vi "Get Data.vi"(8 "error in":errorcluster, 11 "Cfg Dev in":refnum<class "Vaisala.lvclass">) -> (0 "error out":errorcluster, 2 "Data":refnum<class "Data.lvclass">, 3 "Cfg Dev out":refnum<class "Vaisala.lvclass">)   [LabVIEW 2015, in "Vaisala Library.lvlib" / "Vaisala.lvclass"]
uses:
  Vaisala.lvclass
  <vilib>/MSR Consulting, LLC/General Reuse/Session APIs/Serial/Serial Session.lvclass
  Data/Vaisala Data.lvclass
  <vilib>/MSR Consulting, LLC/General Reuse/Data/Data.lvclass
  <vilib>/MSR Consulting, LLC/General Reuse/Session APIs/Session Log/System Log.lvclass
  <vilib>/MSR Consulting, LLC/General Reuse/Session APIs/Serial/Public/Get Data/Get String.vi
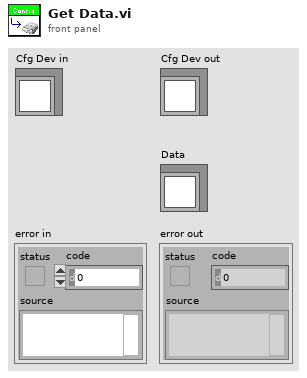
[diagram p1: front panel]
types:
  T1 = typedef "Session - Root.lvclass/Session Handle.ctl" = refnum<data-value>
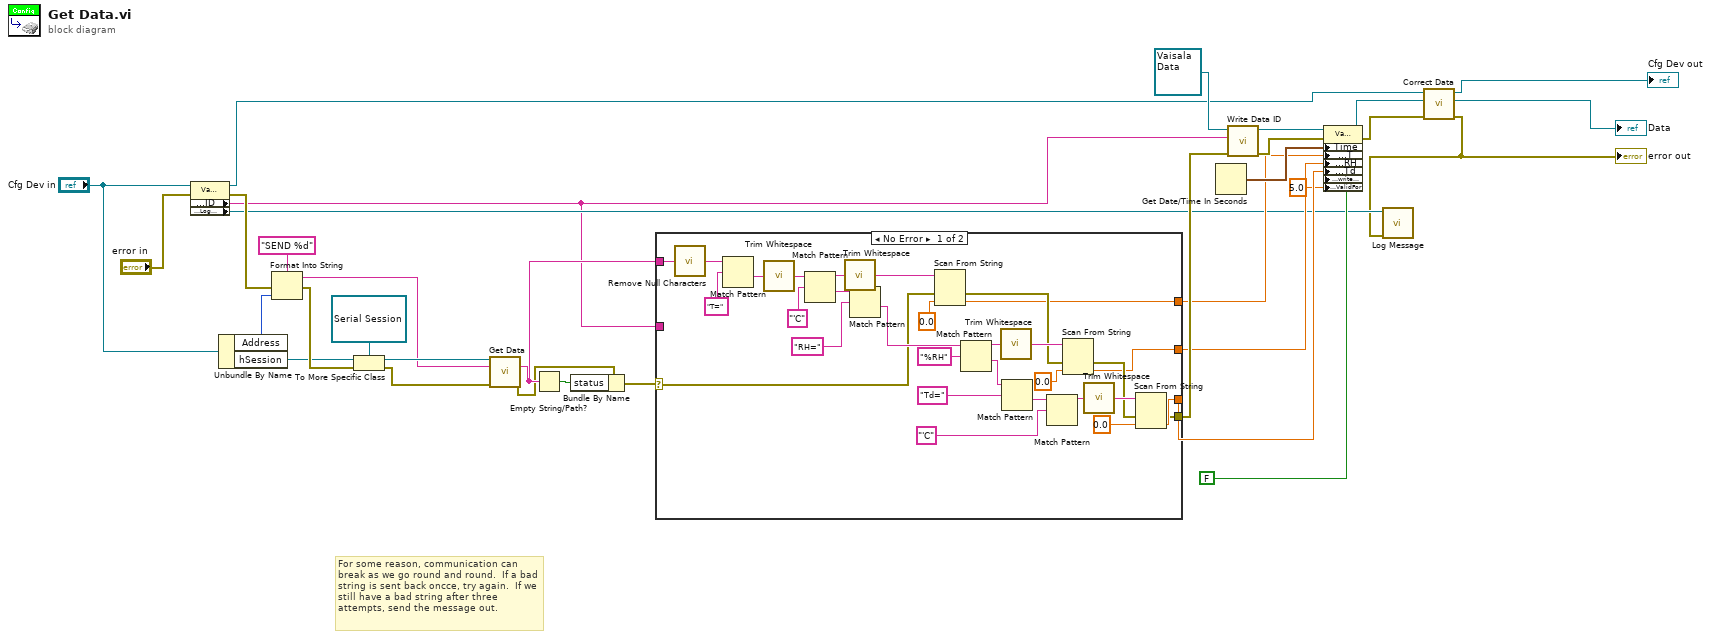
[diagram p0: block diagram]
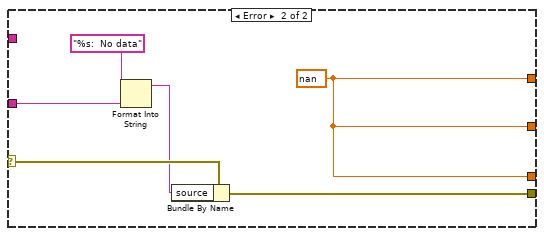
[diagram p2: hidden frame]
diagram:
  # "For some reason, communication can break as we go round and round.  If a bad string is sent back oncce, try again.  If we still have a bad string after three attempts, send the message out."
  n1 = property class="Vaisala.lvclass"(reference="Cfg Dev in", error in="error in") -> (reference out=w10:refnum<class "Vaisala.lvclass">, error out=w19:errorcluster, "Accessors:ID"=w2:string, "Accessors:Log Session"=w12:T1)
  n2 = Unbundle By Name("Cfg Dev in") -> ("Address"=w33:u8, "hSession"=w28:T1)
  n3 = Format Into String(format string="SEND %d", error in=w19, w33) -> (resulting string=w14:string, error out=w29:errorcluster)  [unwired: 1 in]
  n4 = To More Specific Class(target class=refnum<data-value> refnum ("hSession"), reference=w28, error in=w29) -> (specific class reference=w27:refnum<data-value>, error out=w26:errorcluster)
  n5 = call-poly <vilib>:"Get Data.vi"("Session Handle in"=w27, "CMD"=w14, "error in"=w26) -> ("DataOut"=w13:string, "error out"=w5:errorcluster)  [unwired: 10 in, 1 out]
  n6 = Empty String/Path?(string/path=w13) -> (empty?=w4:bool)
  n7 = Bundle By Name(cluster=w5, "status"=w4) -> (w3:errorcluster)
  n8 = case shown="No Error" w3 {
    selector: w3 -> [w34 w66]
    tunnel: [w40 w69] -> w15
    tunnel: [w39 w69] -> w16
    tunnel: [w38 w69] -> w17
    tunnel: [w37 w65] -> w18
    tunnel: w13 -> [w35 _]
    tunnel: w2 -> [_ w67]
    frame No Error {
      n9 = call <vilib>:"Remove Null Characters.vi"("String"=w35) -> ("string"=w36:string)  [unwired: 4 in]
      n10 = Match Pattern(string=w36, regular expression="T=") -> (after substring=w62:string)  [unwired: 1 in, 3 out]
      n11 = call <vilib>:"Trim Whitespace.vi"("string"=w62) -> ("trimmed string"=w61:string)  [unwired: 1 in]
      n12 = Match Pattern(string=w61, regular expression="'C") -> (before substring=w59:string, after substring=w56:string)  [unwired: 1 in, 2 out]
      n13 = call <vilib>:"Trim Whitespace.vi"("string"=w59) -> ("trimmed string"=w58:string)  [unwired: 1 in]
      n14 = Match Pattern(string=w56, regular expression="RH=") -> (after substring=w53:string)  [unwired: 1 in, 3 out]
      n15 = Scan From String(input string=w58, error in=w34, default 1=sgl 0.0 ("output 1")) -> (error out=w42:errorcluster, output 1=w38:sgl)  [unwired: 2 in, 2 out]
      n16 = Match Pattern(string=w53, regular expression="%RH") -> (before substring=w50:string, after substring=w48:string)  [unwired: 1 in, 2 out]
      n17 = call <vilib>:"Trim Whitespace.vi"("string"=w50) -> ("trimmed string"=w51:string)  [unwired: 1 in]
      n18 = Match Pattern(string=w48, regular expression="Td=") -> (after substring=w46:string)  [unwired: 1 in, 3 out]
      n19 = Match Pattern(string=w46, regular expression="'C") -> (before substring=w43:string)  [unwired: 1 in, 3 out]
      n20 = Scan From String(input string=w51, error in=w42, default 1=sgl 0.0 ("output 1")) -> (error out=w41:errorcluster, output 1=w39:sgl)  [unwired: 2 in, 2 out]
      n21 = call <vilib>:"Trim Whitespace.vi"("string"=w43) -> ("trimmed string"=w44:string)  [unwired: 1 in]
      n22 = Scan From String(input string=w44, error in=w41, default 1=sgl 0.0 ("output 1")) -> (error out=w37:errorcluster, output 1=w40:sgl)  [unwired: 2 in, 2 out]
    }
    frame Error {
      w69 = sgl nan ("output 1")
      n23 = Format Into String(format string="%s:  No data", w67) -> (resulting string=w64:string)  [unwired: 2 in, 1 out]
      n24 = Bundle By Name(cluster=w66, "source"=w64) -> (w65:errorcluster)
    }
  }
  n25 = Get Date/Time In Seconds() -> (seconds since 1Jan1904=w31:timestamp)
  n26 = call <vilib>:"Write Data ID.vi"("error in"=w18, "Data ID"=w2, "Data in"=refnum<class "Vaisala Data.lvclass"> refnum ("Vaisala Library.lvlib:Vaisala Data.lvclass")) -> ("error out"=w23:errorcluster, "Data out"=w24:refnum<class "Vaisala Data.lvclass">)  [unwired: 7 in]
  n27 = property class="Vaisala Data"(reference=w24, error in=w23, "Time"=w31, "Accessors:T"=w17, "Accessors:RH"=w16, "Accessors:Td"=w15, "Accessors:write time"=FALSE ("write time"), "Accessors:ValidFor"=5.0 ("ValidFor")) -> (reference out=w9:refnum<class "Vaisala Data.lvclass">, error out=w11:errorcluster)
  n28 = call-dynamic "Correct Data.vi"("error in (no error)"=w11, "Data In"=w9, "Vaisala in"=w10) -> ("error out"=w7:errorcluster, "Data Out"=→"Data":refnum<class "Data.lvclass">, "Vaisala out"=→"Cfg Dev out":refnum<class "Vaisala.lvclass">)  [unwired: 6 in]
  "error out" <- w7
  n29 = call <vilib>:"Log Message.vi"("error in"=w7, "session in"=w12) -> ()  [unwired: 8 in, 2 out]
